vi "Flatten.vi"(6 "FIFO Timestamps":T1, 8 "error in (no error)":errorcluster, 10 "Data":T2[](array[typedef]), 11 "CIFTag in":refnum<class "CIF_NIChn_Fifo_Power.lvclass">) -> (0 "error out":errorcluster, 2 "Data out":T2[](array[typedef]), 3 "CIFTag out":refnum<class "CIF_NIChn_Fifo_Power.lvclass">)   [LabVIEW 2021, in "CIF_NIChn_Fifo_Power.lvclass"]
uses:
  CIF_NIChn_Fifo_Power.lvclass
  D:/dev/Packages/Channel_Manager/src/CIFChannels/CIFChannels.lvclass
  ChannelCommon/typedef/Datatype Waveform.ctl
  ChannelCommon/typedef/TimeStamps.ctl
  CIF_NIChn_Fifo_Power.lvclass/CIF_NIChn_Fifo_Power.ctl
  CIFChannels/CIFChannels.lvclass/CIFChannels.ctl
  <vilib>/CIF Foundation/CIF Utilities/DataTypes/Flatten I64.vi
  ChannelCommon/CIFFIFO/Flatten/Waveform Flatten.vi/be24e584-1bb9-4ddb-b1ad-5fa4498d0a1e.vi
  <vilib>/CIF Foundation/CIF Utilities/DataTypes/Flatten U64.vi
  CIFChannels/Utilities/Create Flattened FIFO Header.vi
  ChannelCommon/CIFFIFO/Flatten/Waveform Flatten.vi/be24e584-1bb9-4ddb-b1ad-5fa4498d0a1e.vi/c28b0ead-42ad-4072-80a2-aca7f2bd7ce3.vi
  ChannelCommon/Utilities/Flatten Header.vi
  CIFChannels/Utilities/Update FIFO Header.vi
  <vilib>/CIF Foundation/CIF Utilities/Time/System Time/Get System Time.vi
  <vilib>/CIF Foundation/CIF Utilities/Time/System Time/LabVIEW Time to TAI Time.vi
  ChannelCommon/ChannelCommon.lvlib
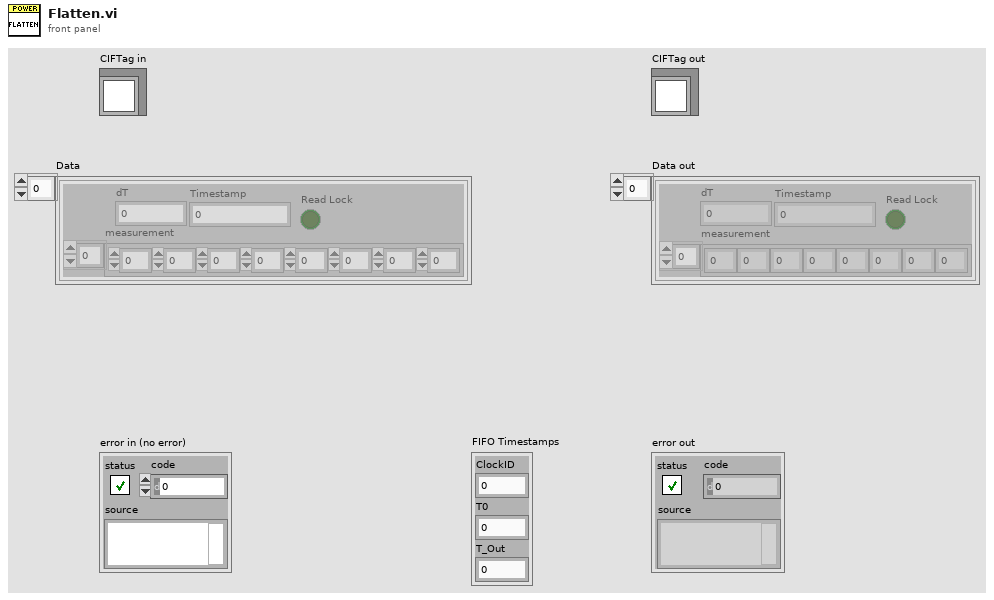
[diagram p1: front panel]
types:
  T1 = typedef "ChannelCommon.lvlib/TimeStamps.ctl" = cluster{"ClockID":u8, "T0":i64, "T_Out":i64}
  T2 = typedef "ChannelCommon.lvlib/Datatype Waveform.ctl" = cluster{"measurement":dbl[], "dT":dbl, "Timestamp":i64, "Read Lock":bool}
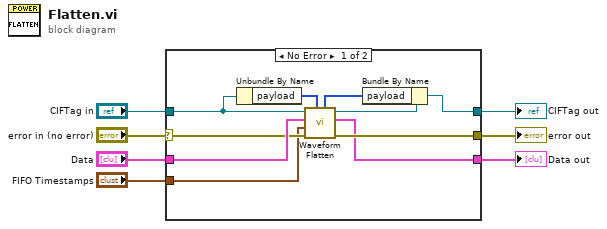
[diagram p0: block diagram]
diagram:
  n1 = case shown="No Error" "error in (no error)" {
    selector: "error in (no error)" -> [w9 w20]
    tunnel: [w17 w20] -> w6
    tunnel: [w16 w19] -> w5
    tunnel: "CIFTag in" -> [w11 w19]
    tunnel: "Data" -> [w15 w18]
    tunnel: [w14 w18] -> w3
    tunnel: "FIFO Timestamps" -> [w8 _]
    frame No Error {
      n2 = Unbundle By Name(w11) -> ("payload"=w13:u8[])
      n3 = call "Waveform Flatten.vi"("payload in"=w13, "error in (no error)"=w9, "FIFO Timestamps"=w8, "Data in"=w15, "CIFChannels in"=w11) -> ("error out"=w17:errorcluster, "Data out"=w14:T2[], "CIFChannels out"=w10:refnum<class "CIF_NIChn_Fifo_Power.lvclass">, "payload out"=w12:u8[])  [unwired: 2 in, 1 out]
      n4 = Bundle By Name(cluster=w10, "payload"=w12) -> (w16:refnum<class "CIF_NIChn_Fifo_Power.lvclass">)
    }
    frame Error {
    }
  }
  "error out" <- w6
  "CIFTag out" <- w5
  "Data out" <- w3
